vi "Frame Done.vi"(8 "Payload Complete":bool, 10 "error in (no error)":errorcluster, 11 "Timeout ms":i32) -> (0 "Done":bool, 2 "error out":errorcluster, 3 "Remaining  Timeout":i32)   [LabVIEW 2020, in "HTTP Server.lvlib" / "WebSocket Client.lvclass"]
uses:
  WebSocket Client.lvclass
  WebSocket Client.lvclass/WebSocket Client.ctl
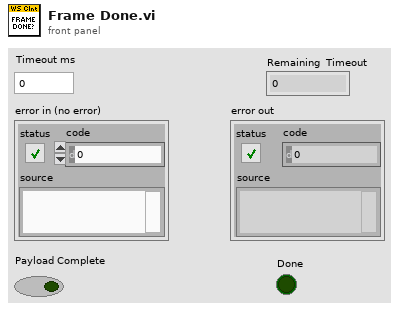
[diagram p1: front panel]
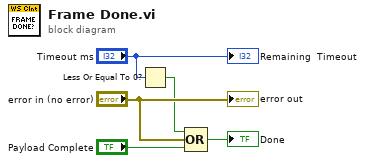
[diagram p0: block diagram]
diagram:
  n1 = Less Or Equal To 0?(x="Timeout ms") -> (x <= 0?=w3:bool)
  n2 = Compound Arithmetic op=OR(w3, "error in (no error)", "Payload Complete") -> (→"Done":bool)
  "Remaining  Timeout" <- "Timeout ms"
  "error out" <- "error in (no error)"
